vi "Resample (constant to constant, complex multi-channel).vi"(5 "anti-aliasing?":bool=TRUE, 6 "FIR filter specifications":T1={"alias rejection (dB)"=120.0, "normalized bandwidth"=0.4536} {"normalized bandwidth" format="%.4f"; "alias rejection (dB)" format="%.2f"}, 7 "reset?":bool, 8 "error in (no error)":errorcluster, 9 "dt":dbl=1.0, 10 "delay":dbl, 11 "X":cdb[][](array[numeric]) format="%#.6g") -> (0 "error out":errorcluster, 2 "t0":dbl, 3 "Y":cdb[][](array[numeric]) format="%#.6g")   [LabVIEW 2017, in "NI_AALPro.lvlib"]
doc: "Resamples input signal <B>X</B> according to <B>delay</B> and <B>dt</B> using an FIR filter implementation. Wire data to the <B>X</B> input to determine the polymorphic instance to use or manually select the instance."
uses:
  NI_AALPro.lvlib
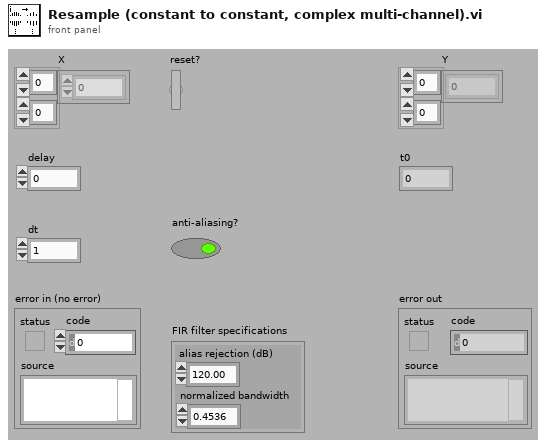
[diagram p1: front panel]
types:
  T1 = cluster{"alias rejection (dB)":dbl, "normalized bandwidth":dbl}
  T2 = cluster{"new sample period":dbl, "Timing Jitter":enum32{"Interpolation", "Rounding"}, "first point location":dbl, "prototype filter":cluster{"h":dbl[], "Max Decimation":i32}}
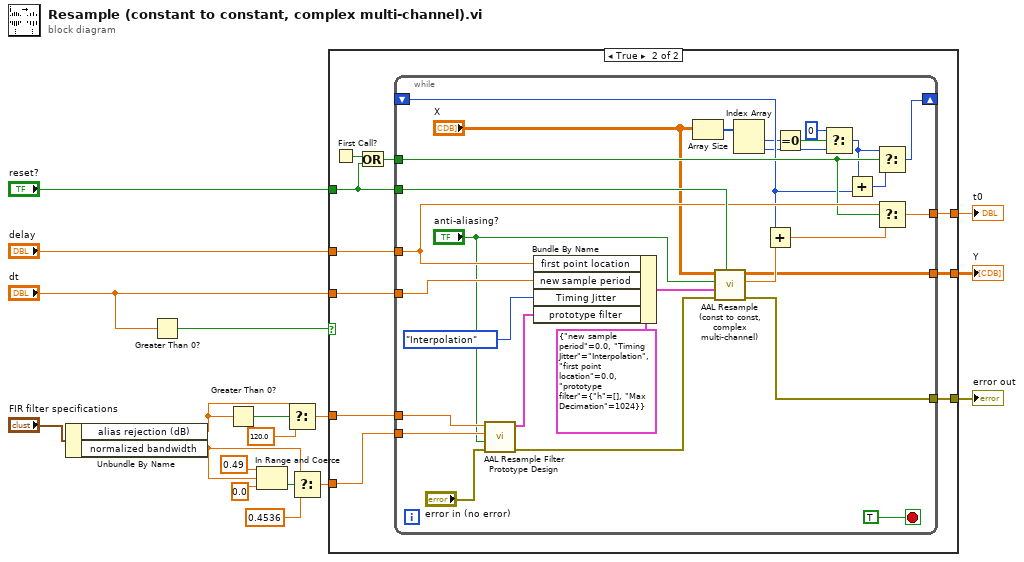
[diagram p0: block diagram]
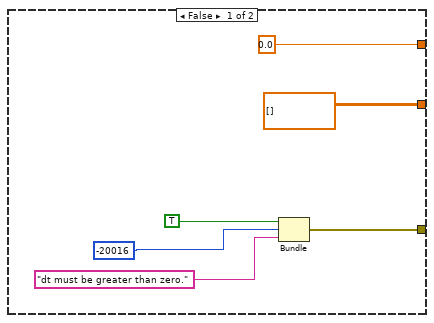
[diagram p2: hidden frame]
diagram:
  n1 = Unbundle By Name("FIR filter specifications") -> ("alias rejection (dB)"=w2:dbl, "normalized bandwidth"=w5:dbl)
  n2 = Greater Than 0?(x="dt") -> (x > 0?=w13:bool)
  n3 = Greater Than 0?(x=w2) -> (x > 0?=w1:bool)
  n4 = In Range and Coerce(upper limit=0.49, x=w5, lower limit=0.0 ("upper limit")) -> (In Range?=w7:bool)  [unwired: 1 out]
  n5 = Select(t=w2, s=w1, f=120.0) -> (s? t:f=w4:dbl)
  n6 = Select(t=w5, s=w7, f=0.4536 ("upper limit")) -> (s? t:f=w3:dbl)
  n7 = case shown="True" w13 {
    tunnel: "dt" -> [_ w32]
    tunnel: "reset?" -> [_ w31]
    tunnel: "delay" -> [_ w30]
    tunnel: [0.0 ("delay") w29] -> w16
    tunnel: [cdb[][] [] ("Y") w28] -> w15
    tunnel: [w23 w27] -> w14
    tunnel: w4 -> [_ w26]
    tunnel: w3 -> [_ w25]
    frame False {
      n8 = Bundle(TRUE, "DtGTZeroErr"=-20016, "dt must be greater than zero.") -> (w23:cluster{bool, "DtGTZeroErr":i32, string})  [unwired: 1 in]
    }
    frame True {
      n9 = First Call?() -> (First Call?: T/F=w34:bool)
      n10 = Or(x=w34, y=w31) -> (x .or. y?=w33:bool)
      n11 = while {
        tunnel: w31 -> [w62]
        tunnel: w30 -> [w53]
        tunnel: w33 -> [w51]
        tunnel: [w55] -> w27
        tunnel: [w52] -> w28
        shift-right: [w48] -> _
        shift-left: _ -> [w45]
        tunnel: [w46] -> w29
        tunnel: w32 -> [w43]
        tunnel: w26 -> [w42]
        tunnel: w25 -> [w41]
        stop <- TRUE stop-if-true
        n12 = call "AAL Resample Filter Prototype Design.vi"("error in (no error)"="error in (no error)", "alias free"="anti-aliasing?", "normalized bandwidth"=w41, "A stop [dB]"=w42) -> ("error out"=w58:errorcluster, "filter prototype"=w59:cluster{"coefficients":dbl[], "factor":i32})  [unwired: 5 in, 1 out]
        n13 = Bundle By Name(cluster=T2 {"new sample period"=0.0, "Timing Jitter"=enum."Interpolation", "first point location"=0.0, "prototype filter"={"h"=[], "Max Decimation"=1024}} ("config"), "first point location"=w53, "new sample period"=w43, "Timing Jitter"=enum32{"Interpolation", "Rounding"}."Interpolation", "prototype filter"=w59) -> (w57:T2)
        n14 = Array Size(array="X") -> (size(s)=w49:i32[])
        n15 = call "AAL Resample (const to const, complex multi-channel).vi"("reset?"=w62, "error in (no error)"=w58, "config"=w57, "anti-aliasing?"="anti-aliasing?", "X"="X") -> ("error out"=w55:errorcluster, "normalized t0"=w54:dbl, "Y"=w52:cdb[][])  [unwired: 4 in]
        n16 = Index Array(array=w49) -> (element #1=w39:i32, element #2=w38:i32)  [unwired: 2 in]
        n17 = Add(x=w45, y=w54) -> (x+y=w47:dbl)
        n18 = Equal To 0?(x=w39) -> (x = 0?=w37:bool)
        n19 = Select(t=0, s=w37, f=w38) -> (s? t:f=w36:i32)
        n20 = Add(x=w36, y=w45) -> (x+y=w44:i32)
        n21 = Select(t=w36, s=w51, f=w44) -> (s? t:f=w48:i32)
        n22 = Select(t=w53, s=w51, f=w47) -> (s? t:f=w46:dbl)
      }
    }
  }
  "t0" <- w16
  "error out" <- w14
  "Y" <- w15
